vi "calc_orientation.vi"(5 "Kx data":cluster{"x":dbl[], "y":dbl[], "z":dbl[]}, 7 "Dx data":cluster{"x":dbl[], "y":dbl[], "z":dbl[]}, 11 "error in":errorcluster) -> (4 "offset":cluster{"x":dbl, "y":dbl, "z":dbl}, 6 "orientation":cluster{"pitch":dbl, "roll":dbl, "yaw":dbl}, 8 "residual":dbl, 10 "orthoganality":dbl, 15 "error out":errorcluster)   [LabVIEW 2011, in "gVision.lvlib"]
uses:
  gVision.lvlib
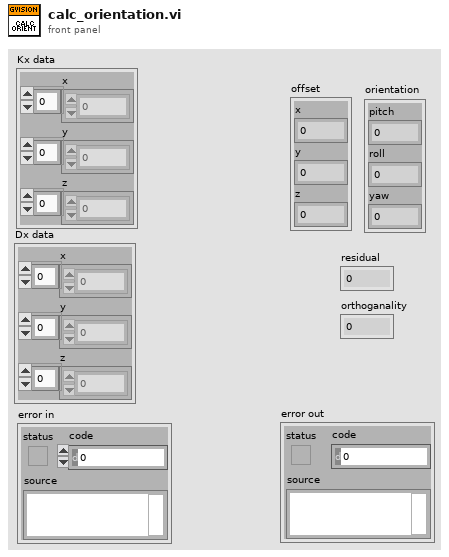
[diagram p1: front panel]
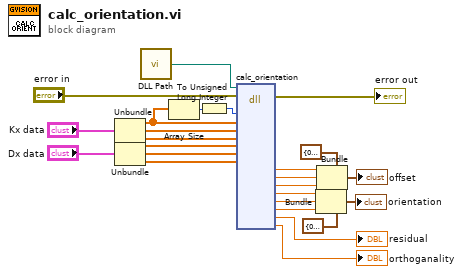
[diagram p0: block diagram]
diagram:
  n1 = Unbundle("Kx data") -> ("x"=w17:dbl[], "y"=w23:dbl[], "z"=w22:dbl[])
  n2 = Unbundle("Dx data") -> ("x"=w20:dbl[], "y"=w19:dbl[], "z"=w18:dbl[])
  n3 = call "DLL Path.vi"() -> ("DLL Path"=w25:path)  [unwired: 5 in]
  n4 = Array Size(array=w17) -> (size(s)=w16:i32)
  n5 = To Unsigned Long Integer(number=w16) -> (unsigned 32bit integer=w15:u32)
  n6 = dll-call lib="?" fn="calc_orientation"(path in=w25, error in="error in", "n"=w15, "Kx_in"=w17, "Ky_in"=w23, "Kz_in"=w22, "Dx_in"=w20, "Dy_in"=w19, "Dz_in"=w18) -> (error out=→"error out":errorcluster, "offset_x"=w13:dbl, "offset_y"=w12:dbl, "offset_z"=w11:dbl, "pitch"=w8:dbl, "roll"=w7:dbl, "yaw"=w6:dbl, "residual"=→"residual":dbl, "orthoganality"=→"orthoganality":dbl)  [unwired: 17 in, 1 out]
  n7 = Bundle(cluster=cluster{"pitch":dbl, "roll":dbl, "yaw":dbl} {"pitch"=0.0, "roll"=0.0, "yaw"=0.0}, "pitch"=w8, "roll"=w7, "yaw"=w6) -> (→"orientation":cluster{"pitch":dbl, "roll":dbl, "yaw":dbl})
  n8 = Bundle(cluster=cluster{"x":dbl, "y":dbl, "z":dbl} {"x"=0.0, "y"=0.0, "z"=0.0}, "x"=w13, "y"=w12, "z"=w11) -> (→"offset":cluster{"x":dbl, "y":dbl, "z":dbl})
